vi "Launch Valve.vi"(4 "Stop Action (Close)":T1=enum."Close", 5 "Start Action (Open)":T1, 6 "SHV":refnum<k21>[](array[refnum]), 7 "Name":string, 8 "error in (no error)":errorcluster, 9 "StateQ":refnum<queue>, 10 "Interlock Chain":refnum<class "Interlock Chain.lvclass">, 11 "cRIO-CO2 in":refnum<class "cRIO-CO2.lvclass">) -> (0 "error out":errorcluster, 3 "cRIO-CO2 out":refnum<class "cRIO-CO2.lvclass">)   [LabVIEW 2015, in "cRIO-Carbondioxide.lvlib" / "cRIO-CO2.lvlib" / "cRIO-CO2.lvclass"]
uses:
  cRIO-CO2.lvclass
  Interlocks/Interlock Chain/Interlock Chain.lvclass
  Valve/Action.ctl
  <vilib>/ActorFramework/Actor/Actor.lvclass
  cRIO-CO2.lvclass/cRIO-CO2.ctl
  cRIO-CO2 Messages/Log Message Msg/Log Message Msg.lvclass/Log Message Msg.ctl
  <vilib>/ActorFramework/Message Enqueuer/Message Enqueuer.lvclass/Message Enqueuer.ctl
  <vilib>/ActorFramework/Message Enqueuer/Enqueue.vi
  <vilib>/ActorFramework/Message Priority Queue/Priority Enqueue.vi
  <vilib>/ActorFramework/Message Enqueuer/Message Enqueuer.lvclass
  cRIO-CO2 Messages/Log Message Msg/Log Message Msg.lvclass
  Valve/Valve.lvclass
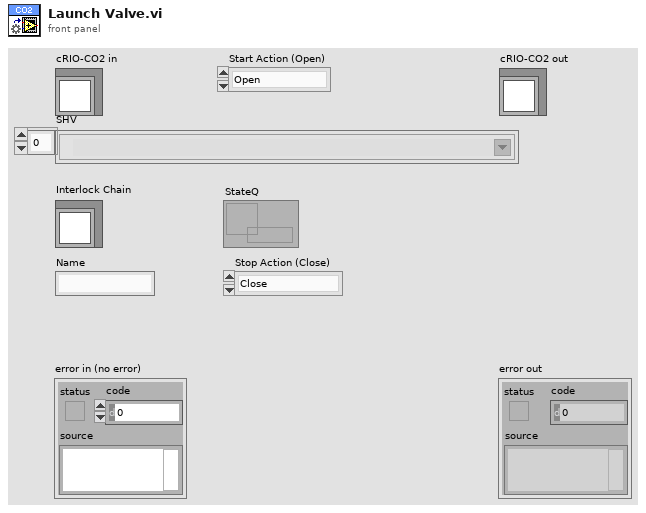
[diagram p1: front panel]
types:
  T1 = typedef "Action.ctl" = enum16{"Open", "Close", "None"}
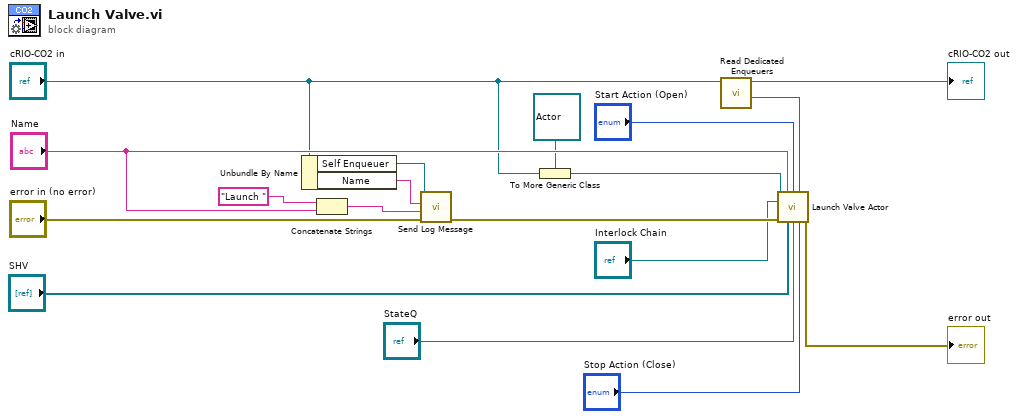
[diagram p0: block diagram]
diagram:
  n1 = Unbundle By Name("cRIO-CO2 in") -> ("Self Enqueuer"=w16:refnum<class "Message Enqueuer.lvclass">, "Name"=w17:string)
  n2 = Concatenate Strings("Launch " ("String"), "Name") -> (w13:string)
  n3 = call "Send Log Message.vi"("error in (no error)"="error in (no error)", "String"=w13, "Source Name"=w17, "Message Enqueuer"=w16) -> ("error out"=w15:errorcluster)  [unwired: 6 in, 1 out]
  n4 = To More Generic Class(target class=refnum<class "Actor.lvclass"> refnum ("Caller Actor in"), reference="cRIO-CO2 in") -> (generic class reference=w7:refnum<class "Actor.lvclass">)
  n5 = call "Read Dedicated Enqueuers.vi"("cRIO-CO2 in"="cRIO-CO2 in") -> ("Qs.DedicatedEnQrs"=w2:refnum<queue>, "cRIO-CO2 out"=→"cRIO-CO2 out":refnum<class "cRIO-CO2.lvclass">)  [unwired: 7 in, 2 out]
  n6 = call "Launch Valve Actor.vi"("Caller Actor in"=w7, "Name"="Name", "Start Action (Open)"="Start Action (Open)", "DedicatedEnQrs"=w2, "Interlock Chain"="Interlock Chain", "error in (no error)"=w15, "SHV"="SHV", "StateQ"="StateQ", "Stop Action (Close)"="Stop Action (Close)") -> ("error out"=→"error out":errorcluster)  [unwired: 5 in, 1 out]
